vi "RPED Set.vi"() -> ()   [LabVIEW 2017]
uses:
  <vilib>/Rock Robotics/WPI/DriverStation/WPI_DriverStationRobotMode2.ctl
  RPED Control Type.ctl
  RPED Globals.vi
  Robot Global Data.vi
panel:
  out "error out 2":errorcluster
  out "error out":errorcluster
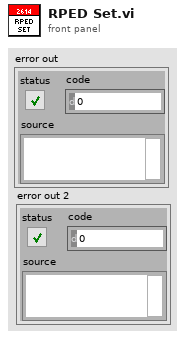
[diagram p1: front panel]
types:
  T1 = typedef "RPED Control Type.ctl" = enum16{"No Op", "Left Manual", "Right Manual", "Time", "Left", "Right", "Left_Distance", "Right_Distance"}
  T2 = typedef "WPI_DriverStationRobotMode2.ctl" = enum16{"Autonomous Disabled", "Autonomous Enabled", "Teleop Disabled", "Teleop Enabled", "Disconnected", "Finish", "Test Disabled", "Test Enabled", "Emergency Stopped"}
  T3 = typedef "RPED Notifier.ctl" = cluster{"RPED Control Type":T1, "Step":i32, "Left Forward":bool, "Right Forward":bool, "Parameter 1":dbl, "Parameter 2":dbl, "Parameter 3":dbl, "RPED Notifier":refnum<notifier>, "Left Back":bool, "Right Back":bool, "Right":bool, "Left":bool}
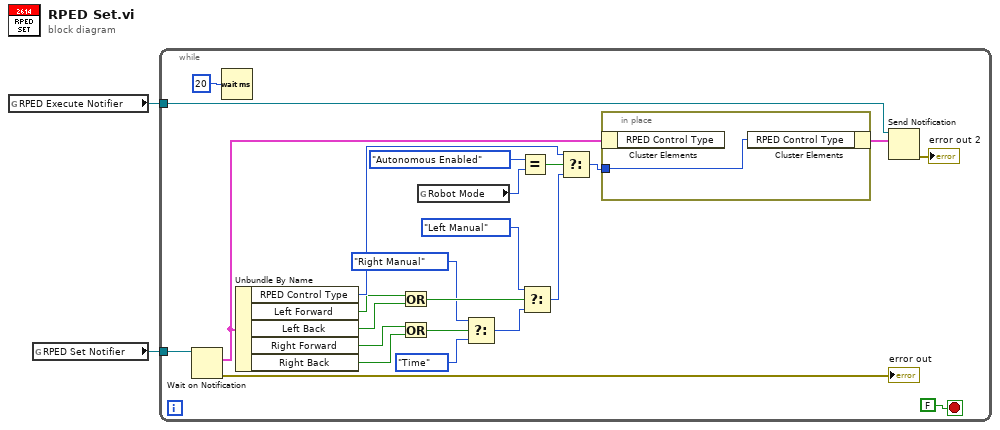
[diagram p0: block diagram]
diagram:
  n1 = global read "RPED Globals.vi" "RPED Execute Notifier"() -> (w1:refnum<notifier>)
  n2 = global read "RPED Globals.vi" "RPED Set Notifier"() -> (w2:refnum<notifier>)
  n3 = while {
    tunnel: w2 -> [w23]
    tunnel: w1 -> [w22]
    stop <- FALSE stop-if-true
    n4 = Wait on Notification(notifier=w23) -> (notification=w21:T3, error out=→"error out":errorcluster)  [unwired: 3 in, 2 out]
    n5 = Wait (ms)(milliseconds to wait=u32 20) -> ()  [unwired: 1 out]
    n6 = Unbundle By Name(w21) -> ("RPED Control Type"=w17:T1, "Left Forward"=w12:bool, "Left Back"=w11:bool, "Right Forward"=w9:bool, "Right Back"=w8:bool)
    n7 = Or(x=w12, y=w11) -> (x .or. y?=w13:bool)
    n8 = Or(x=w9, y=w8) -> (x .or. y?=w10:bool)
    n9 = global read "Robot Global Data.vi" "Robot Mode"() -> (w19:T2)
    n10 = Select(t=RPED_Control_Type."Right Manual", s=w10, f=RPED_Control_Type."Time") -> (s? t:f=w16:T1)
    n11 = Equal?(x=WPI_DriverStationRobotMode2."Autonomous Enabled", y=w19) -> (x = y?=w20:bool)
    n12 = Select(t=RPED_Control_Type."Left Manual", s=w13, f=w16) -> (s? t:f=w15:T1)
    n13 = Select(t=w17, s=w20, f=w15) -> (s? t:f=w14:T1)
    n14 = in-place {
      in-place-border: w14 -> [w27]
      n15 = in-place-cluster #1(w21) -> ()  [unwired: 1 out]
      n16 = in-place-cluster #1("RPED Control Type"=w27) -> (w24:T3)
    }
    n17 = Send Notification(notification=w24, notifier=w22) -> (error out=→"error out 2":errorcluster)  [unwired: 1 in, 1 out]
  }
